vi "Launcher.vi"() -> ()   [LabVIEW 2019]
uses:
  Queues/Queues FGV Action.ctl
  User Event/Controls/UE Abort Action.ctl
  Queues/Queues.lvlib
  Controller/Controller.lvlib
  UI/UIs.lvlib
  Camera/Andor/Andor.lvlib
  IO/sbRIO9623/sbRIO9623.lvlib
  Laser/Coherent/Coherent.lvlib
  LED/LED.lvlib
  Motion/Allmotion/Allmotion.lvlib
  Selection Valve/IDEX/IDEX.lvlib
  Syringe Pump/NE-500/NE-500.lvlib
  Fluidic Process/Fluidic Process.lvlib
  Image/Image.lvlib
panel:
  in  "Error In":errorcluster
  out "Error Out":errorcluster
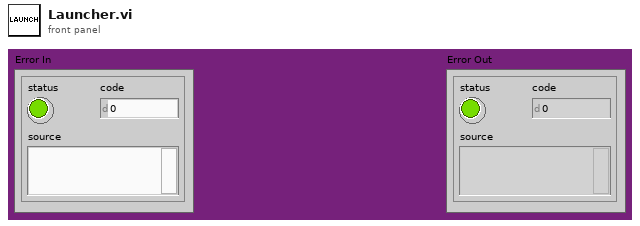
[diagram p1: front panel]
types:
  T1 = typedef "Queues.lvlib/Queues FGV Action.ctl" = enum16{"Obtain Queues", "Release Queues"}
  T2 = typedef "UE Abort Action.ctl" = enum16{"Create", "Get", "Destroy"}
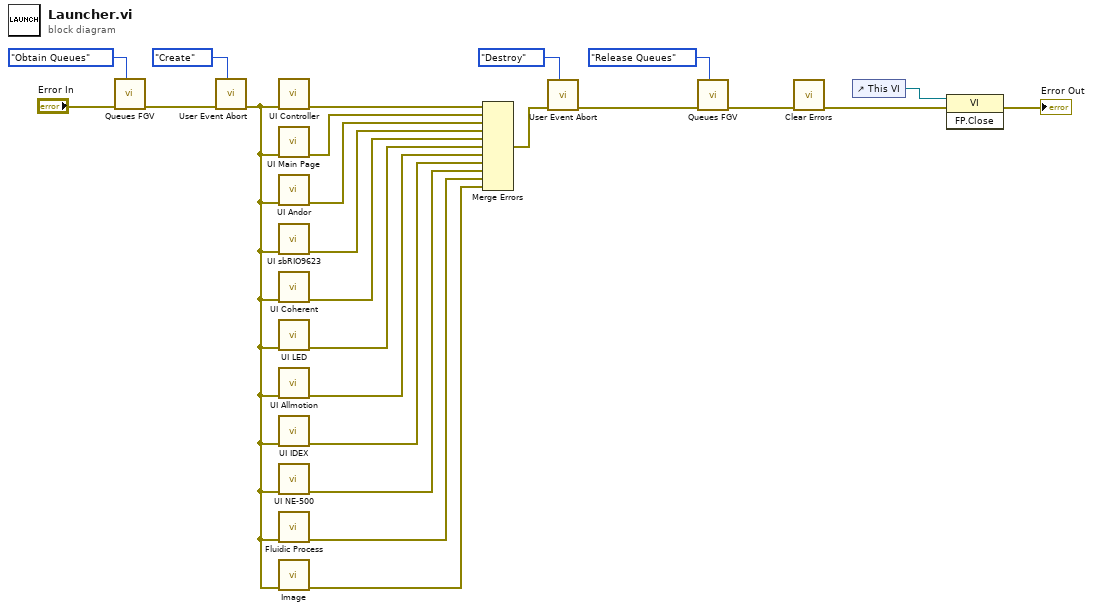
[diagram p0: block diagram]
diagram:
  n1 = call "Queues FGV.vi"("Action"=Queues_FGV_Action."Obtain Queues", "Error In"="Error In") -> ("Error Out"=w22:errorcluster)  [unwired: 9 in]
  n2 = call "User Event Abort.vi"("Action"=UE_Abort_Action."Create", "Error In"=w22) -> ("Error Out"=w14:errorcluster)  [unwired: 8 in, 1 out]
  n3 = call "UI Controller.vi"("Error In"=w14) -> ("Error Out"=w18:errorcluster)  [unwired: 10 in]
  n4 = call "UI Main Page.vi"("error in"=w14) -> ("error out"=w17:errorcluster)  [unwired: 10 in]
  n5 = call "UI Andor.vi"("error in"=w14) -> ("error out"=w13:errorcluster)  [unwired: 10 in]
  n6 = call "UI sbRIO9623.vi"("error in"=w14) -> ("error out"=w12:errorcluster)  [unwired: 10 in]
  n7 = call "UI Coherent.vi"("error in"=w14) -> ("error out"=w11:errorcluster)  [unwired: 10 in]
  n8 = call "UI LED.vi"("error in"=w14) -> ("error out"=w10:errorcluster)  [unwired: 10 in]
  n9 = call "UI Allmotion.vi"("error in"=w14) -> ("error out"=w9:errorcluster)  [unwired: 10 in]
  n10 = call "UI IDEX.vi"("error in"=w14) -> ("error out"=w8:errorcluster)  [unwired: 10 in]
  n11 = call "UI NE-500.vi"("error in"=w14) -> ("error out"=w7:errorcluster)  [unwired: 10 in]
  n12 = call "Fluidic Process.vi"("error in"=w14) -> ("error out"=w6:errorcluster)  [unwired: 10 in]
  n13 = call "Image.vi"("error in"=w14) -> ("error out"=w5:errorcluster)  [unwired: 10 in]
  n14 = Merge Errors(w18, w17, w13, w12, w11, w10, w9, w8, w7, w6, w5) -> (w16:errorcluster)
  n15 = call "User Event Abort.vi"("Action"=UE_Abort_Action."Destroy", "Error In"=w16) -> ("Error Out"=w15:errorcluster)  [unwired: 8 in, 1 out]
  n16 = call "Queues FGV.vi"("Action"=Queues_FGV_Action."Release Queues", "Error In"=w15) -> ("Error Out"=w2:errorcluster)  [unwired: 9 in]
  n17 = call <vilib>:"Clear Errors.vi"("error in (no error)"=w2) -> ("error out"=w1:errorcluster)  [unwired: 5 in, 1 out]
  n18 = control-ref of="This VI"() -> (w4:refnum<vi>)
  n19 = invoke class="VI" method="FP.Close"(reference=w4, error in=w1) -> (error out=→"Error Out":errorcluster)  [unwired: 1 in, 2 out]
